vi "calibrateEvent.vi"(8 "error in (no error)":errorcluster, 11 "RfRamp in":refnum<class "RfRamp.lvclass">) -> (0 "error out":errorcluster, 3 "RfRamp out":refnum<class "RfRamp.lvclass">)   [LabVIEW 2009, in "Tools.lvlib" / "Scripting.lvlib" / "RfRamp.lvclass"]
uses:
  RfRamp.lvclass
  Rf Event/rf.lvclass
  RfRamp.lvclass/RfRamp.ctl
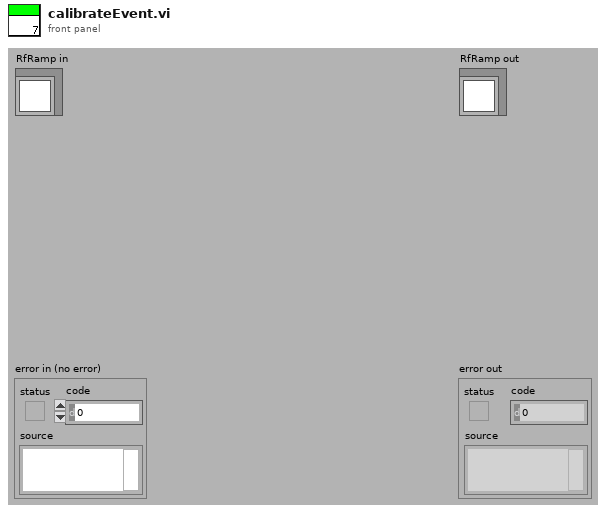
[diagram p1: front panel]
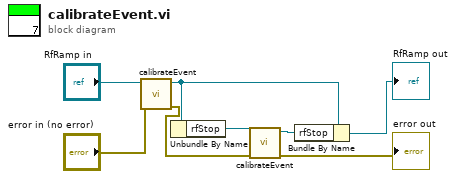
[diagram p0: block diagram]
diagram:
  n1 = call-parent "calibrateEvent.vi"("error in (no error)"="error in (no error)", "rf in"="RfRamp in") -> ("error out"=w1:errorcluster, "rf out"=w5:refnum<class "RfRamp.lvclass">)  [unwired: 8 in]
  n2 = Unbundle By Name(w5) -> ("rfStop"=w6:refnum<class "rf.lvclass">)
  n3 = call-parent "calibrateEvent.vi"("error in (no error)"=w1, "rf in"=w6) -> ("error out"=→"error out":errorcluster, "rf out"=w3:refnum<class "rf.lvclass">)  [unwired: 8 in]
  n4 = Bundle By Name(cluster=w5, "rfStop"=w3) -> (→"RfRamp out":refnum<class "RfRamp.lvclass">)
